vi "InsertIntoArrayCluster.vi"(10 "CH2":T2={"PID Gains"={"proportional gain (Kc)"=1.0, "integral gain (Kc*Ts/Ti)"=0.1, "derivative gain (Kc*Td/Ts)"=0.0}, "Output Range"={"output high"=1.0, "output low"=-1.0}}, 11 "CH1":T2={"PID Gains"={"proportional gain (Kc)"=1.0, "integral gain (Kc*Ts/Ti)"=0.1, "derivative gain (Kc*Td/Ts)"=0.0}, "Output Range"={"output high"=1.0, "output low"=-1.0}}) -> (1 "OR Low array":dbl[](array[numeric]), 2 "OR High array":dbl[](array[numeric]), 3 "PID Gains array":T1(array[cluster]))   [LabVIEW 2014]
uses:
  controls/Control ConfigurationSam.ctl
panel:
  # "This one only works for doubles"
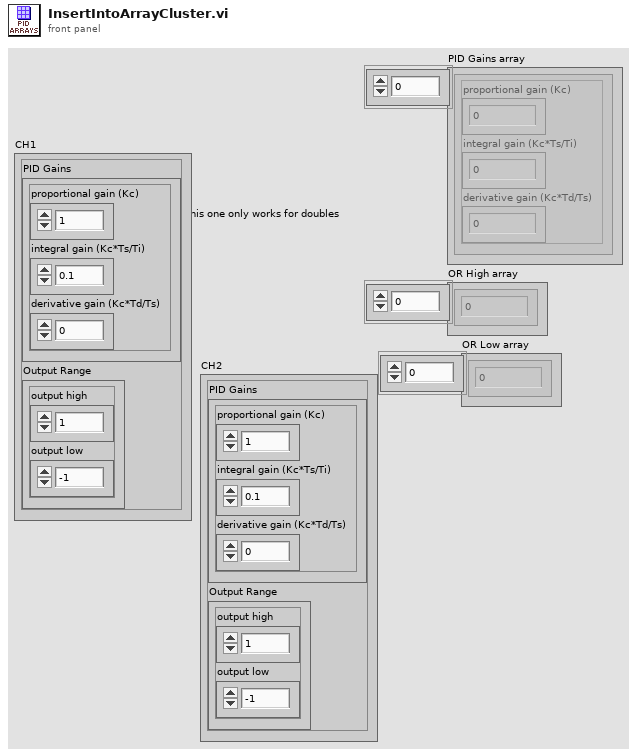
[diagram p1: front panel]
types:
  T1 = cluster{"proportional gain (Kc)":dbl, "integral gain (Kc*Ts/Ti)":dbl, "derivative gain (Kc*Td/Ts)":dbl}[]
  T2 = typedef "Control ConfigurationSam.ctl" = cluster{"PID Gains":cluster{"proportional gain (Kc)":dbl, "integral gain (Kc*Ts/Ti)":dbl, "derivative gain (Kc*Td/Ts)":dbl}, "Output Range":cluster{"output high":dbl, "output low":dbl}}
  T3 = cluster{"proportional gain (Kc)":dbl, "integral gain (Kc*Ts/Ti)":dbl, "derivative gain (Kc*Td/Ts)":dbl}
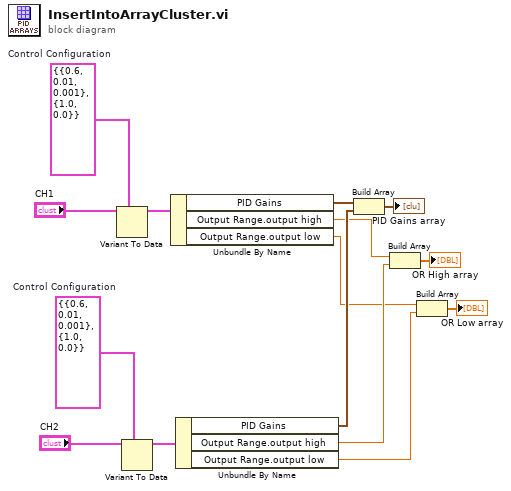
[diagram p0: block diagram]
diagram:
  w12 = T2 {"PID Gains"={"proportional gain (Kc)"=0.6, "integral gain (Kc*Ts/Ti)"=0.01, "derivative gain (Kc*Td/Ts)"=0.001}, "Output Range"={"output high"=1.0, "output low"=0.0}}  # Control Configuration
  w15 = T2 {"PID Gains"={"proportional gain (Kc)"=0.6, "integral gain (Kc*Ts/Ti)"=0.01, "derivative gain (Kc*Td/Ts)"=0.001}, "Output Range"={"output high"=1.0, "output low"=0.0}}  # Control Configuration
  n1 = Variant To Data(type=w15, Variant="CH1") -> (data=w11:T2)  [unwired: 1 in, 1 out]
  n2 = Variant To Data(type=w12, Variant="CH2") -> (data=w10:T2)  [unwired: 1 in, 1 out]
  n3 = Unbundle By Name(w11) -> ("PID Gains"=w9:T3, "Output Range.output high"=w6:dbl, "Output Range.output low"=w4:dbl)
  n4 = Unbundle By Name(w10) -> ("PID Gains"=w8:T3, "Output Range.output high"=w5:dbl, "Output Range.output low"=w3:dbl)
  n5 = Build Array(w9, w8) -> (→"PID Gains array":T1)
  n6 = Build Array(w6, w5) -> (→"OR High array":dbl[])
  n7 = Build Array(w4, w3) -> (→"OR Low array":dbl[])
